vi "PH_VacuumControl.evt Set Lagarithmic MT.vi"(0 "i ref in":refnum<vi>, 1 "Instance":string="N/A", 2 "MT Logarithmic?":bool, 5 "error in (no error)":errorcluster) -> (14 "i ref out":refnum<vi>, 19 "error out":errorcluster)   [LabVIEW 2014, in "PH_VacuumControl.lvlib"]
doc: "This VI sets the trend Channel"
uses:
  PH_VacuumControl.lvlib
  CSCore/CSSystem/CoreLib/CoreLib.short 2 byte array.vi
  CSCore/CSSystem/CoreLib/CoreLib.lvlib
  CSCore/BaseProcess/BaseProcess.lvlib
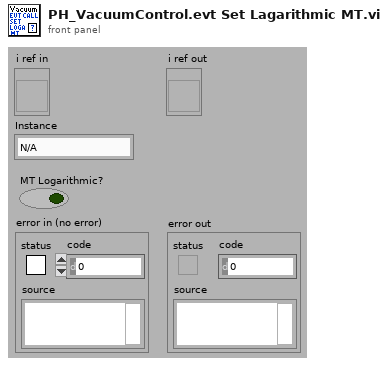
[diagram p1: front panel]
types:
  T1 = typedef "CoreDefs.rawDataType.ctl" = i8[]
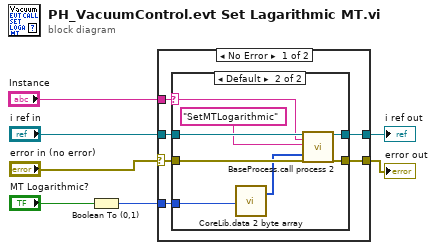
[diagram p0: block diagram]
diagram:
  n1 = Boolean To (0,1)(Boolean="MT Logarithmic?") -> (0, 1=w1:i16)
  n2 = case shown="No Error" "error in (no error)" {
    selector: "error in (no error)" -> [w8 w24]
    tunnel: [w13 w25] -> w7
    tunnel: [w12 w24] -> w6
    tunnel: "i ref in" -> [w11 w25]
    tunnel: "Instance" -> [w10 _]
    tunnel: w1 -> [w9 _]
    frame No Error {
      n3 = case shown="Default" w10 {
        selector: w10 -> [_ w19]
        tunnel: [w15 w23] -> w13
        tunnel: [w14 w22] -> w12
        tunnel: w11 -> [w15 w21]
        tunnel: w8 -> [w14 w20]
        tunnel: w9 -> [_ w17]
        frame "N/A" {
        }
        frame Default {
          n4 = call-poly "CoreLib.data 2 byte array.vi"("i16"=w17) -> ("byteArray out"=w16:T1)  [unwired: 18 in]
          n5 = call "BaseProcess.call process 2.vi"("i ref in"=w21, "Object"=w19, "Selector"="SetMTLogarithmic", "Data"=w16, "error in (no error)"=w20) -> ("i ref out"=w23:refnum<vi>, "error out"=w22:errorcluster)  [unwired: 13 in]
        }
      }
    }
    frame Error {
    }
  }
  "error out" <- w6
  "i ref out" <- w7
